vi "Initialize.vi"(6 "optional":variant, 8 "error in":errorcluster, 11 "Category in":refnum<class "Category.lvclass">) -> (0 "error out":errorcluster, 3 "Node*":refnum<data-value>)   [LabVIEW 2013, in "Category.lvclass"]
doc: "Initializes a xceDataNode."
uses:
  Category.lvclass
  xCE/xceNode/xceNode.lvclass
  xCE/xceDataNode/xceDataNode.lvclass
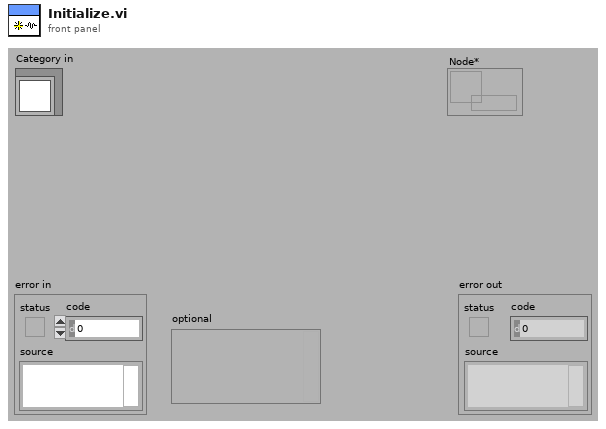
[diagram p1: front panel]
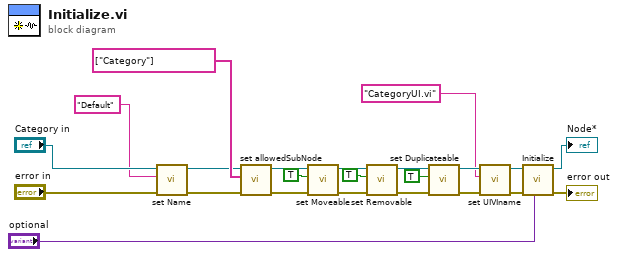
[diagram p0: block diagram]
diagram:
  n1 = call "set Name.vi"("error in (no error)"="error in", "Name"="Default", "xceDataNode in"="Category in") -> ("error out"=w2:errorcluster, "xceDataNode out"=w3:refnum<class "Category.lvclass">)  [unwired: 7 in]
  n2 = call "set allowedSubNode.vi"("error in (no error)"=w2, "Allowed subNode[]"=string[] ["Category"], "xceDataNode in"=w3) -> ("error out"=w18:errorcluster, "xceDataNode out"=w19:refnum<class "Category.lvclass">)  [unwired: 7 in]
  n3 = call "set Moveable.vi"("error in (no error)"=w18, "Moveable"=TRUE, "xceDataNode in"=w19) -> ("error out"=w15:errorcluster, "xceDataNode out"=w16:refnum<class "Category.lvclass">)  [unwired: 7 in]
  n4 = call "set Removable.vi"("error in (no error)"=w15, "Removable"=TRUE, "xceDataNode in"=w16) -> ("error out"=w12:errorcluster, "xceDataNode out"=w13:refnum<class "Category.lvclass">)  [unwired: 7 in]
  n5 = call "set Duplicateable.vi"("error in (no error)"=w12, "Duplicateable"=TRUE, "xceDataNode in"=w13) -> ("error out"=w9:errorcluster, "xceDataNode out"=w10:refnum<class "Category.lvclass">)  [unwired: 7 in]
  n6 = call "set UIVIname.vi"("error in (no error)"=w9, "UI VI name"="CategoryUI.vi", "xceDataNode in"=w10) -> ("error out"=w6:errorcluster, "xceDataNode out"=w7:refnum<class "Category.lvclass">)  [unwired: 7 in]
  n7 = call-parent "Initialize.vi"("optional"="optional", "error in"=w6, "xceDataNode in"=w7) -> ("error out"=→"error out":errorcluster, "Node*"=→"Node*":refnum<data-value>)  [unwired: 7 in]
